vi "Days elapsed from year(0000).vi"(11 "Date/Time":string="12-Mar-2018 11:55:33") -> (3 "No of days passed from the date(00/00/0000)":i32)   [LabVIEW 2019]
doc: "Days elapsed from year 0000"
panel:
  out "No of leap years from the year 0000":u64
  out "End Day":i32
  out "End Year":i32
  out "No of days elapsed \nbefore that month":i32
  out "End Month":i32
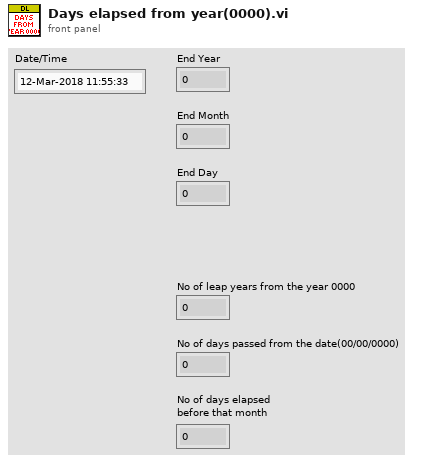
[diagram p1: front panel]
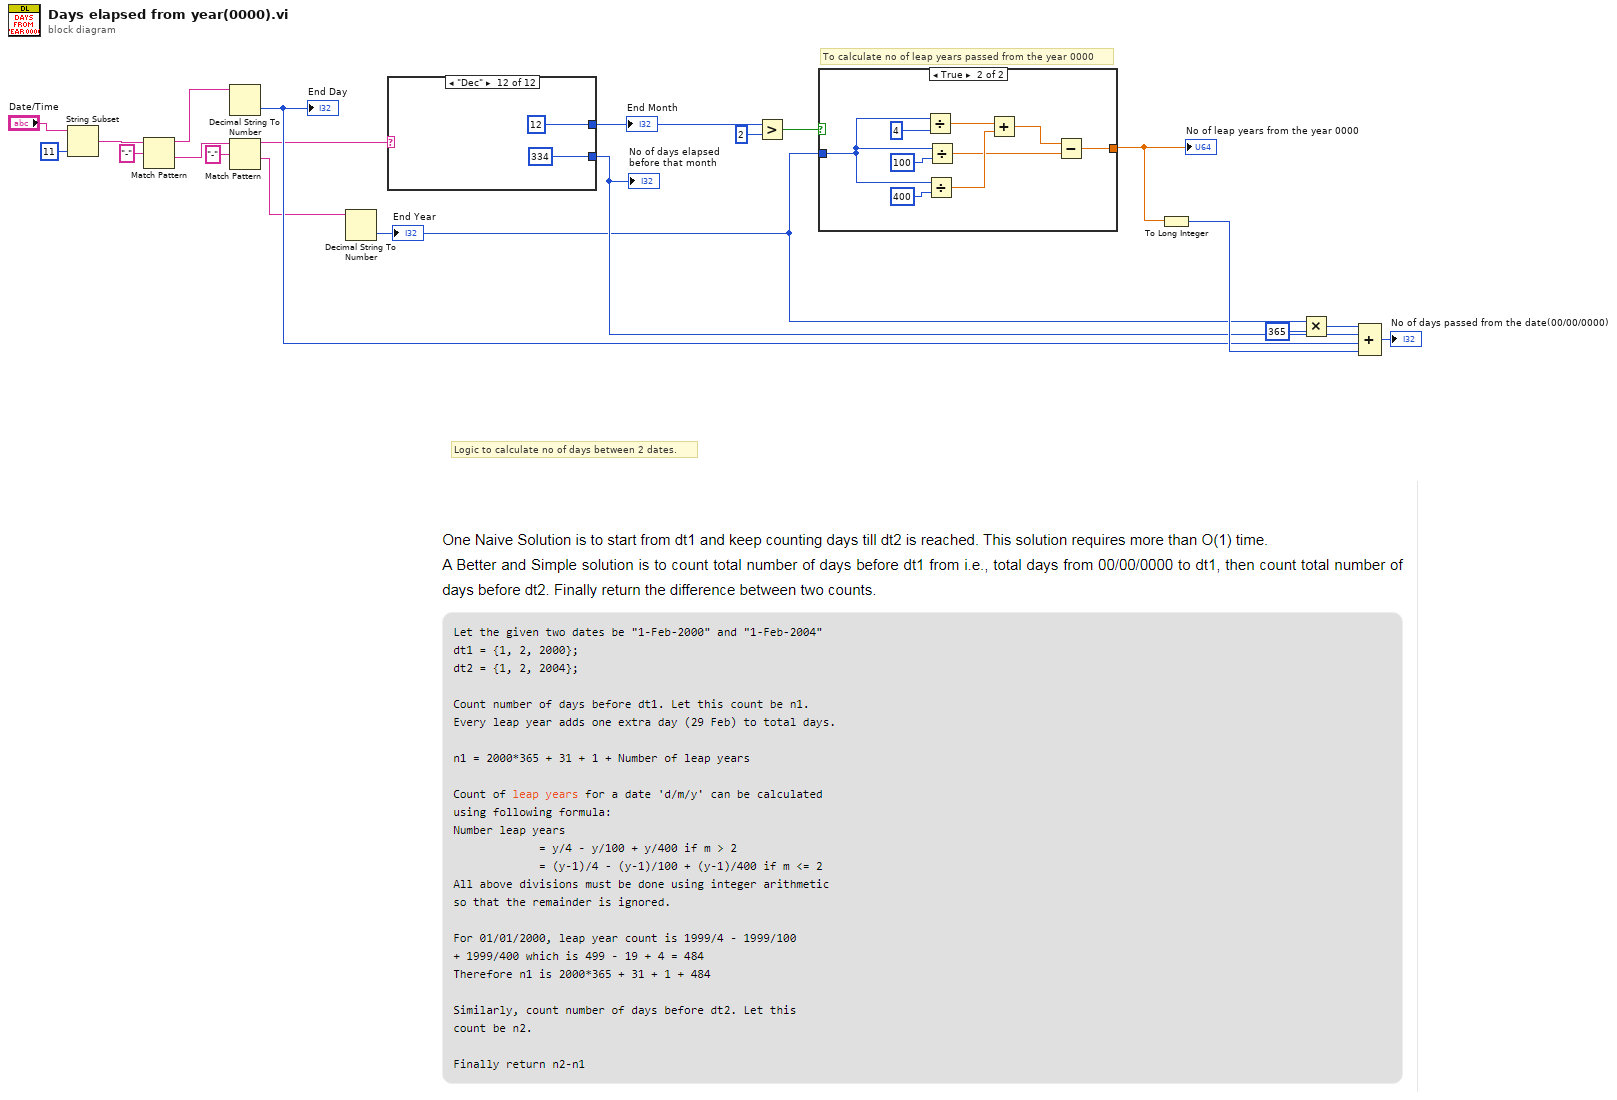
[diagram p0: block diagram]
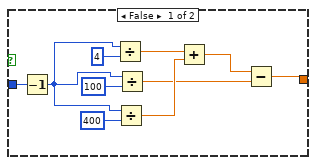
[diagram p2: hidden frame]
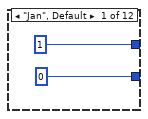
[diagram p3: hidden frame]
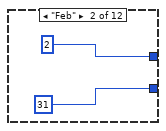
[diagram p4: hidden frame]
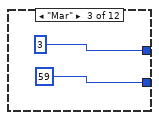
[diagram p5: hidden frame]
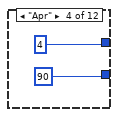
[diagram p6: hidden frame]
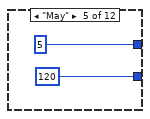
[diagram p7: hidden frame]
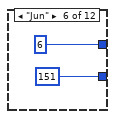
[diagram p8: hidden frame]
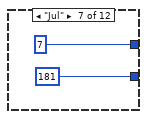
[diagram p9: hidden frame]
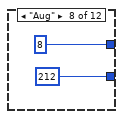
[diagram p10: hidden frame]
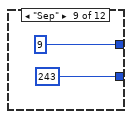
[diagram p11: hidden frame]
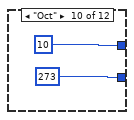
[diagram p12: hidden frame]
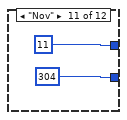
[diagram p13: hidden frame]
diagram:
  # "Logic to calculate no of days between 2 dates."
  # "To calculate no of leap years passed from the year 0000"
  n1 = String Subset(string="Date/Time", length (rest)=11 ("length (rest)")) -> (substring=w2:string)  [unwired: 1 in]
  n2 = Match Pattern(string=w2, regular expression="-") -> (before substring=w8:string, after substring=w4:string)  [unwired: 1 in, 2 out]
  n3 = Decimal String To Number(string=w8) -> (number=w16:i32)  [unwired: 2 in, 1 out]
  "End Day" <- w16
  n4 = Match Pattern(string=w4, regular expression="-") -> (before substring=w6:string, after substring=w7:string)  [unwired: 1 in, 2 out]
  n5 = Decimal String To Number(string=w7) -> (number=w12:i32)  [unwired: 2 in, 1 out]
  "End Year" <- w12
  n6 = case shown="\"Dec\"" w6 {
    tunnel: [1 2 3 4 5 6 7 8 9 10 11 12] -> w9
    tunnel: [0 31 59 90 120 151 181 212 243 273 304 334] -> w15
    frame "Jan", Default {
    }
    frame "Feb" {
    }
    frame "Mar" {
    }
    frame "Apr" {
    }
    frame "May" {
    }
    frame "Jun" {
    }
    frame "Jul" {
    }
    frame "Aug" {
    }
    frame "Sep" {
    }
    frame "Oct" {
    }
    frame "Nov" {
    }
    frame "Dec" {
    }
  }
  "End Month" <- w9
  "No of days elapsed \nbefore that month" <- w15
  n7 = Greater?(x=w9, y=2) -> (0:w10:bool)
  n8 = case shown="True" w10 {
    tunnel: w12 -> [w47 w60]
    tunnel: [w48 w55] -> w17
    frame False {
      n9 = Decrement(x=w47) -> (x-1=w46:i32)
      n10 = Divide(x=w46, y=4) -> (x/y=w52:dbl)
      n11 = Divide(x=w46, y=400) -> (x/y=w51:dbl)
      n12 = Divide(x=w46, y=100) -> (x/y=w49:dbl)
      n13 = Add(x=w52, y=w51) -> (x+y=w50:dbl)
      n14 = Subtract(x=w50, y=w49) -> (x-y=w48:dbl)
    }
    frame True {
      n15 = Divide(x=w60, y=4) -> (x/y=w59:dbl)
      n16 = Divide(x=w60, y=400) -> (x/y=w58:dbl)
      n17 = Divide(x=w60, y=100) -> (x/y=w56:dbl)
      n18 = Add(x=w59, y=w58) -> (x+y=w57:dbl)
      n19 = Subtract(x=w57, y=w56) -> (x-y=w55:dbl)
    }
  }
  "No of leap years from the year 0000" <- w17
  n20 = To Long Integer(number=w17) -> (32bit integer=w18:i32)
  n21 = Multiply(x=w12, y=365) -> (x*y=w14:i32)
  n22 = Compound Arithmetic op=ADD(w14, w15, w16, w18) -> (→"No of days passed from the date(00/00/0000)":i32)
